vi "Read VISA.vi"(8 "error in (no error)":errorcluster, 10 "VISA Refnum in":refnum<visa-resource-name>, 11 "NXP in":refnum<class "NXP.lvclass">) -> (0 "error out":errorcluster, 1 "Serial Response":string, 2 "VISA resource name out":refnum<visa-resource-name>, 3 "NXP out":refnum<class "NXP.lvclass">)   [LabVIEW 2020, in "NXP.lvclass"]
uses:
  NXP.lvclass
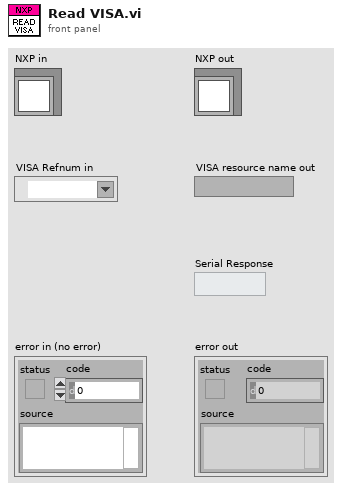
[diagram p1: front panel]
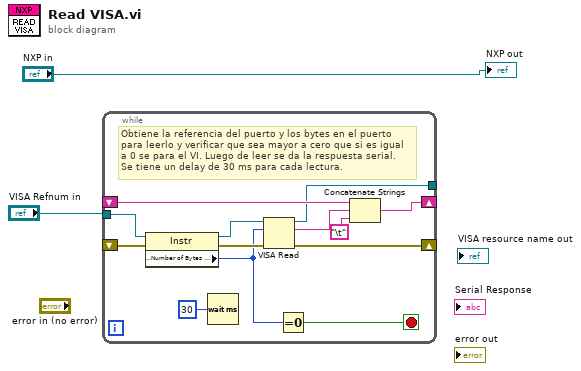
[diagram p0: block diagram]
diagram:
  n1 = while {
    tunnel: "VISA Refnum in" -> [w15]
    shift-right: [w14] -> _
    shift-left: _ -> [w13]
    shift-right: [w9] -> _
    shift-left: _ -> [w10]
    tunnel: [w5] -> _
    stop <- w6 stop-if-true
    # "Obtiene la referencia del puerto y los bytes en el puerto\npara leerlo y verificar que sea mayor a cero que si es igual\na 0 se para el VI. Luego de leer se da la respuesta serial.\nSe tiene un delay de 30 ms para cada lectura."
    n2 = property class="Instr"(reference=w15, error in=w13) -> (reference out=w11:refnum<visa-resource-name>, error out=w12:errorcluster, "Serial Settings:Number of Bytes at Serial Port"=w7:u32)
    n3 = Wait (ms)(milliseconds to wait=u32 30) -> ()  [unwired: 1 out]
    n4 = VISA Read(VISA resource name=w11, byte count=w7, error in (no error)=w12) -> (VISA resource name out=w5:refnum<visa-resource-name>, read buffer=w4:string, error out=w14:errorcluster)  [unwired: 1 out]
    n5 = Equal To 0?(x=w7) -> (x = 0?=w6:bool)
    n6 = Concatenate Strings(w10, w4, "\t") -> (w9:string)
  }
  "NXP out" <- "NXP in"
